vi "Read ctl.vi"(8 "error in (no error)":errorcluster, 11 "TEC in":refnum<class "TEC.lvclass">) -> (0 "error out":errorcluster, 2 "ctl":cluster{"p":dbl, "i":dbl, "d":dbl}, 3 "TEC out":refnum<class "TEC.lvclass">)   [LabVIEW 2015, in "Generic TEC.lvlib" / "TEC.lvclass"]
uses:
  TEC.lvclass
  TEC.lvclass/TEC.ctl
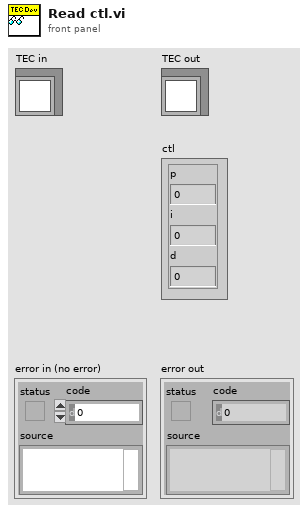
[diagram p1: front panel]
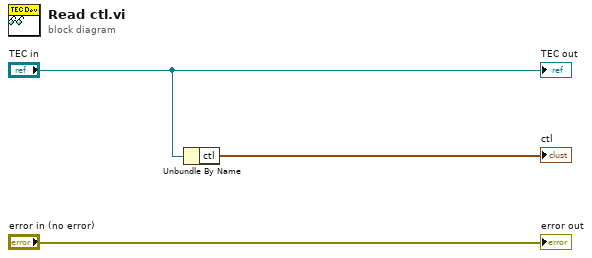
[diagram p0: block diagram]
diagram:
  n1 = Unbundle By Name("TEC in") -> ("ctl"=→"ctl":cluster{"p":dbl, "i":dbl, "d":dbl})
  "error out" <- "error in (no error)"
  "TEC out" <- "TEC in"
